vi "Taiko_TaggedValueListToStrArray.vi"(11 "TaggedValueList":T2 {"Tag" format="%x" items=["NONE"=0, "Locked"=16, "SoftLock"=17, "KeyLock"=18, "Class_IV_Lock"=20, "Interlock"=24, "LaserMode"=32, "LDH_PulsePowerTable"=33, "TriggerMode"=48, "TriggerLevelRaw"=64, "TriggerLevelRawLoLimit"=65, "TriggerLevelRawHiLimit"=66, "TriggerLevel"=72, "TriggerLevelLoLimit"=73, "TriggerLevelHiLimit"=74, "FastGate"=80, "FastGateImp"=96, "SlowGate"=112, "TargetTempRaw"=144, "TargetTempRawLoLimit"=145, "TargetTempRawHiLimit"=146, "CurrentTempRaw"=148, "CaseTempRaw"=149, "TargetTemp"=152, "TargetTempLoLimit"=153, "TargetTempHiLimit"=154, "CurrentTemp"=156, "CaseTemp"=157, "TempScale"=159, "Frequency"=168, "FrequencyLoLimit"=169, "FrequencyHiLimit"=170, "PulsePowerRaw"=176, "PulsePowerRawLoLimit"=177, "PulsePowerRawHiLimit"=178, "PulsePowerPermille"=180, "PulseShape"=181, "PulsePower"=184, "PulsePowerLoLimit"=185, "PulsePowerHiLimit"=186, "PulsePowerNanowatt"=188, "PulsePowerVoltage"=190, "PulseEnergy"=191, "CwPowerRaw"=192, "CwPowerRawLoLimit"=193, "CwPowerRawHiLimit"=194, "CwPowerPermille"=196, "CwPower"=200, "CwPowerLoLimit"=201, "CwPowerHiLimit"=202, "CwPowerMicroWatt"=204, "BurstLen"=208, "BurstPeriod"=224, "LDH_Fan"=240, "UI_Exclusive"=256]}) -> (2 "ValList":string[](array[string]), 3 "TagList":string[](array[string]))   [LabVIEW 2017]
uses:
  _lib/PDLM/pdlm_lib_x86_x64_UIThread.llb/PDLM_TaggedValueList.ctl
  _lib/PDLM/pdlm_lib_x86_x64_UIThread.llb/PDLM_TaggedValue.ctl
  _lib/PDLM/pdlm_lib_x86_x64_UIThread.llb/PDLM_Tag.ctl
  _lib/PDLM/pdlm_lib_x86_x64_UIThread.llb/PDLM_ScaleID.ctl
panel:
  out "ScaleID":T1
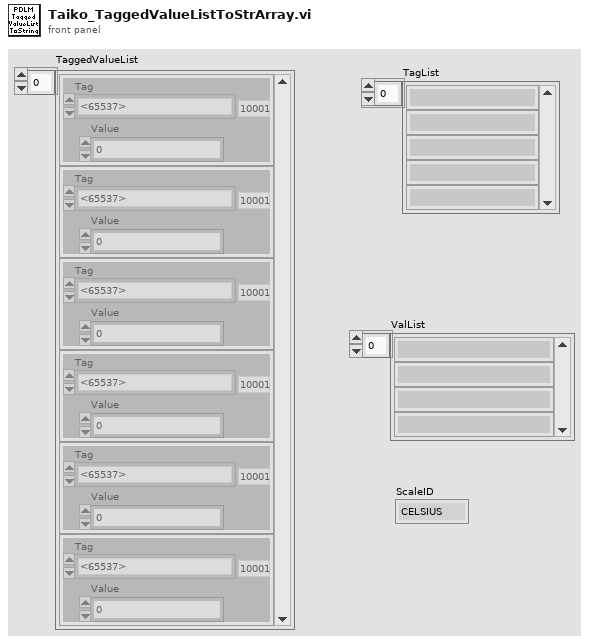
[diagram p1: front panel]
types:
  T1 = typedef "PDLM_ScaleID.ctl" = enum32{"CELSIUS", "FAHRENHEIT", "KELVIN"}
  T2 = typedef "PDLM_TaggedValueList.ctl" = T3[]
  T3 = typedef "PDLM_TaggedValue.ctl" = cluster{"Tag":T4, "Value":u32}
  T4 = typedef "PDLM_Tag.ctl" = u32
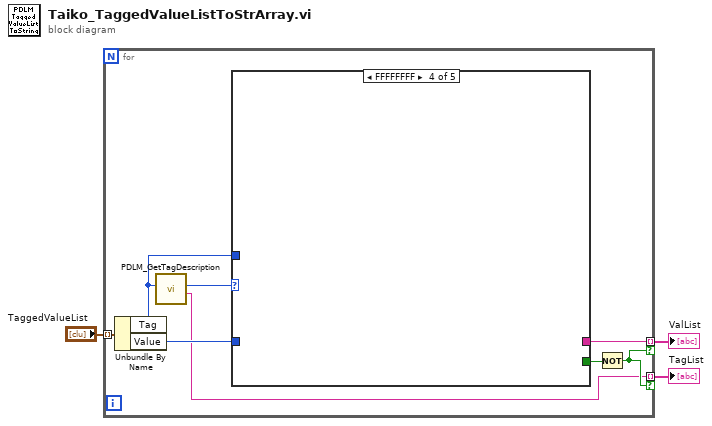
[diagram p0: block diagram]
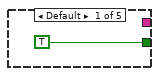
[diagram p2: hidden frame]
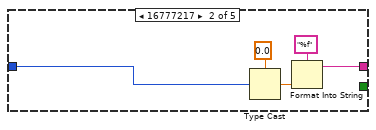
[diagram p3: hidden frame]
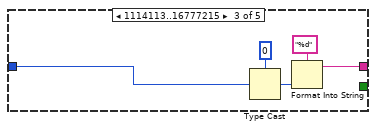
[diagram p4: hidden frame]
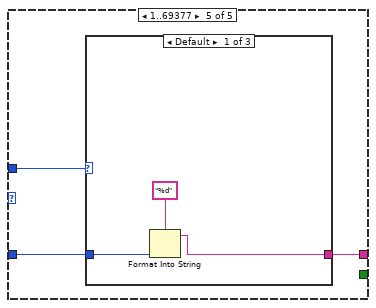
[diagram p5: hidden frame]
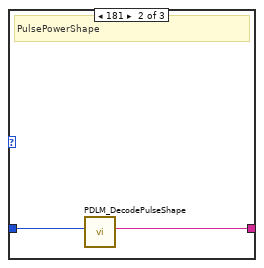
[diagram p6: hidden frame]
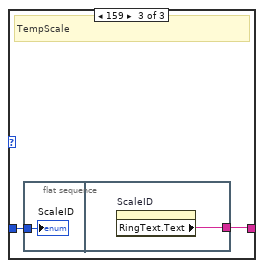
[diagram p7: hidden frame]
diagram:
  n1 = for {
    tunnel: "TaggedValueList" -> [w11] mode=indexing
    tunnel: [w8] -> w2 mode=indexing if=w7
    tunnel: [w6] -> w1 mode=indexing if=w7
    n2 = Unbundle By Name(w11) -> ("Tag"=w4:T4, "Value"=w10:u32)
    n3 = call "PDLM_GetTagDescription.vi"("Tag"=w4) -> ("Name"=w6:string, "TypeCode"=w5:u32)  [unwired: 7 in, 2 out]
    n4 = case shown="FFFFFFFF" w5 {
      tunnel: w10 -> [_ w13 w22 _ w24]
      tunnel: [TRUE _ _ _ _] -> w9
      tunnel: [_ w14 w18 _ w23] -> w8
      tunnel: w4 -> [_ _ _ _ w25]
      frame Default {
      }
      frame 16777217 {
        n5 = Type Cast(type=sgl 0.0, x=w13) -> (*(type *) &x=w16:sgl)
        n6 = Format Into String(format string="%f", w16) -> (resulting string=w14:string)  [unwired: 2 in, 1 out]
      }
      frame 1114113..16777215 {
        n7 = Type Cast(type=0, x=w22) -> (*(type *) &x=w20:i32)
        n8 = Format Into String(format string="%d", w20) -> (resulting string=w18:string)  [unwired: 2 in, 1 out]
      }
      frame -1 {
      }
      frame 1..69377 {
        n9 = case shown="Default" w25 {
          tunnel: w24 -> [w27 w30 w32]
          tunnel: [w26 w29 w31] -> w23
          frame Default {
            n10 = Format Into String(format string="%d", w27) -> (resulting string=w26:string)  [unwired: 2 in, 1 out]
          }
          frame 181 {
            # "PulsePowerShape"
            n11 = call "PDLM_DecodePulseShape.vi"("shape"=w30) -> ("Buffer"=w29:string)  [unwired: 8 in, 2 out]
          }
          frame 159 {
            # "TempScale"
            n12 = flat-sequence {
              tunnel: w32 -> [w33]
              tunnel: [w34] -> w31
              frame #0 {
                "ScaleID" <- w33
              }
              frame #1 {
                n13 = property on="ScaleID" class="Enum (strict)"() -> ("RingText.Text"=w34:string)  [unwired: 2 in, 2 out]
              }
            }
          }
        }
      }
    }
    n14 = Not(x=w9) -> (.not. x?=w7:bool)
  }
  "ValList" <- w2
  "TagList" <- w1
